vi "SafetySystem.vi"() -> ()   [LabVIEW 2018]
uses:
  <vilib>/Platform/TimedLoop/XDataNode/timing_clust.ctl
  <vilib>/Platform/TimedLoop/XDataNode/nitl_modes.ctl
  <vilib>/Platform/TimedLoop/XDataNode/wakeup.ctl
  <vilib>/Modbus/slave/Create Slave Instance (TCP).vi
  <vilib>/Modbus/slave/Modbus Slave.lvclass
  <vilib>/Platform/TimedLoop/XDataNode/XDataNode.xnode
  <vilib>/Platform/TimedLoop/XDataNode/XDNodeRunTimeDep.lvlib
panel:
  out "SIS-10SDV501":bool
  out "SIS-10SDV502":bool
  out "SIS-10SDV500":bool
  out "SIS-10TI101":dbl
  out "SIS-10AI301":dbl
  out "SIS-10LI202":dbl
  out "SIS-10LI201":dbl
  in  "stop":bool
  out "TX-SIS-BPCS-ARRAY":bool[](array[boolean])
  out "BPCS-SIM-TX-ARRAY":dbl[](array[numeric])
  out "SIM-SIS-RX-ARRAY":dbl[](array[numeric])
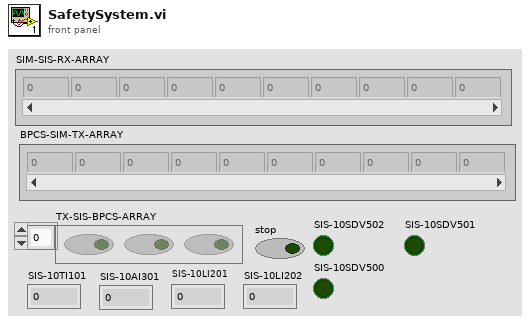
[diagram p1: front panel]
types:
  T1 = typedef "XDNodeRunTimeDep.lvlib/timing_clust.ctl" = cluster{"Expected End [f-1]":u64, "Actual End [f-1]":u64, "Finished Late? [f-1]":bool, "Expected End [i-1]":u64, "Actual End [i-1]":u64, "Finished Late? [i-1]":bool, "Expected Start [i]":u64, "Actual Start [i]":u64, "Expected Start [f]":u64, "Actual Start [f]":u64, "Source Name":string, "Structure Name":string, "Period":i64, "Deadline":i64, "Offset":i64, "Start":i64, "Priority":i32, "Timeout":i32, "Mode":T2, "Wakeup Reason":T3, "Error":errorcluster, "Source Type":string, "Secondary Source Type":string, "Global End Time":u64, "Global Start Time":u64, "Frame Duration":u64, "Iteration Duration":u64, "Assigned CPU":i32, "I/O Scan Engine Mode":u32}
  T2 = typedef "XDNodeRunTimeDep.lvlib/nitl_modes.ctl" = enum32{"No Change", "Process missed periods, maintain original phase", "Discard missed periods, maintain original phase", "Process missed periods, ignore original phase", "Discard missed periods, ignore original phase"}
  T3 = typedef "XDNodeRunTimeDep.lvlib/wakeup.ctl" = enum32{"Normal", "Aborted", "Asynchronous wakeup", "Timing source error", "Timed loop error", "Timeout"}
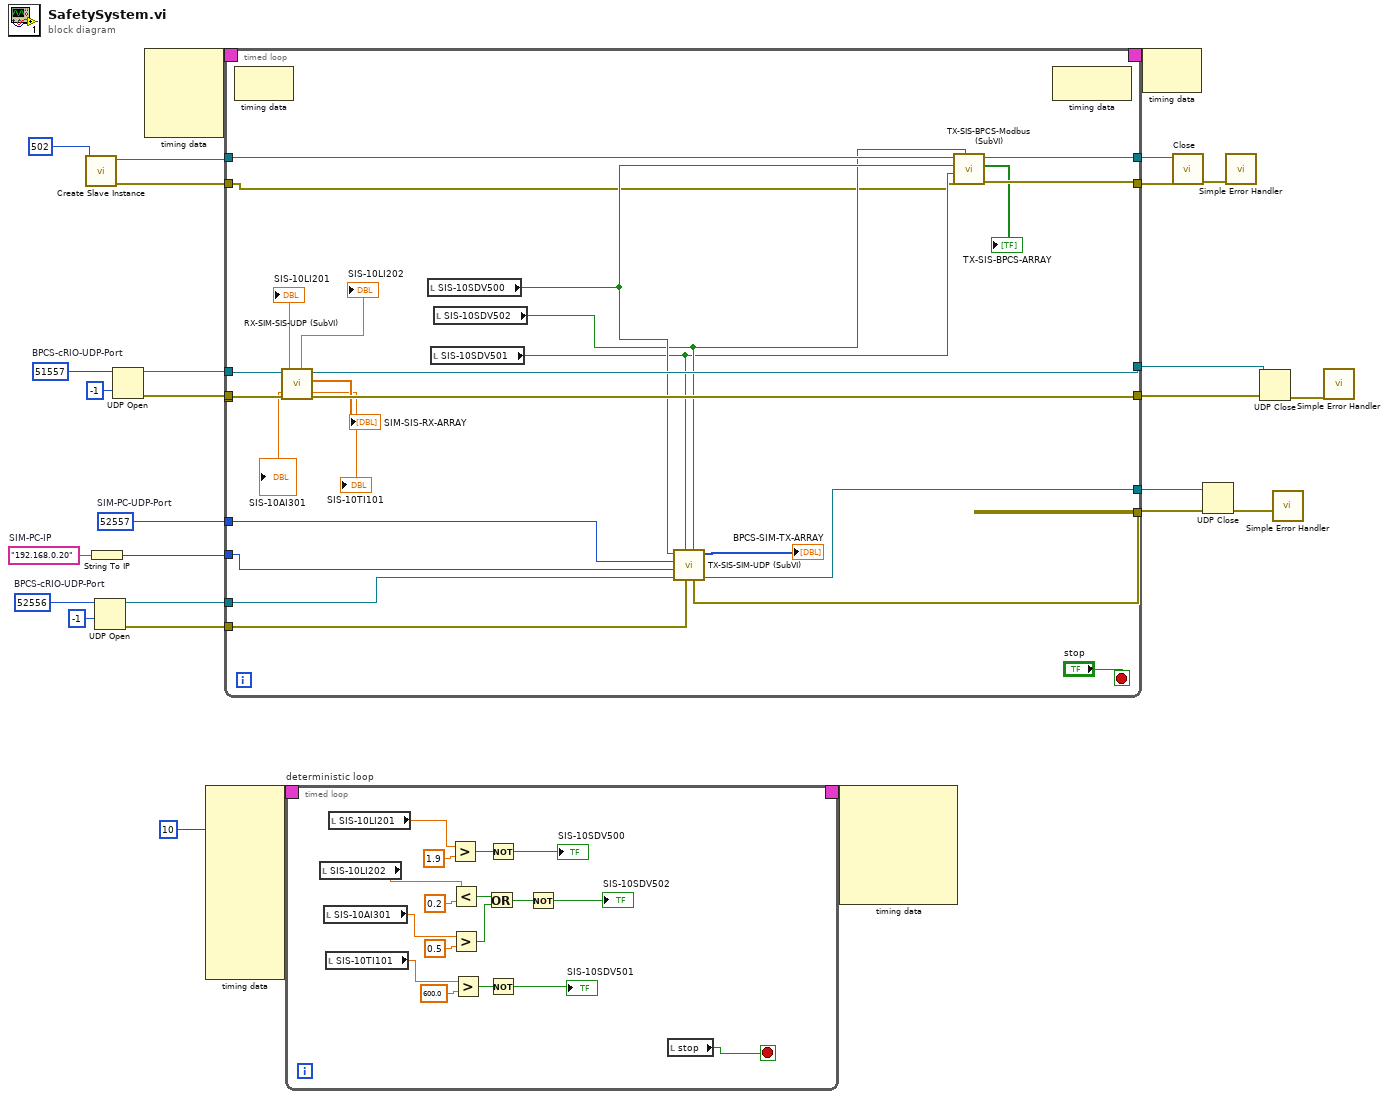
[diagram p0: block diagram]
diagram:
  w18 = u16 52556  # BPCS-cRIO-UDP-Port
  w16 = u16 52557  # SIM-PC-UDP-Port
  w19 = "192.168.0.20"  # SIM-PC-IP
  w25 = u16 51557  # BPCS-cRIO-UDP-Port
  n1 = call-poly <vilib>:"Create Slave Instance.vi"("port (502)"=u16 502) -> ("error out"=w8:errorcluster, "TCP slave instance"=w9:refnum<class "Modbus Slave.lvclass">)  [unwired: 9 in]
  n2 = String To IP(1:w19) -> (0:w15:u32)
  n3 = UDP Open(9:-1 ("timeout ms (25000)"), 11:w18) -> (port=w14:refnum<k16>, 0:w13:errorcluster)  [unwired: 3 in, 1 out]
  n4 = UDP Open(9:-1 ("timeout ms (25000)"), 11:w25) -> (port=w24:refnum<k16>, 0:w23:errorcluster)  [unwired: 3 in, 1 out]
  n5 = node-c288() -> (w28:T1)  [unwired: 4 in]
  n6 = node-c288 ("Input Node")(i64 10 ("Period")) -> (w4:T1)  [unwired: 9 in]
  n7 = timed-loop {
    timing: w28 -> [_]
    timing-out: [_] -> w27
    tunnel: w24 -> [w53]
    tunnel: [w52] -> _
    tunnel: w23 -> [w52]
    tunnel: [w51] -> w21
    tunnel: [w50] -> w20
    tunnel: w16 -> [w40]
    tunnel: w15 -> [w39]
    tunnel: w14 -> [w44]
    tunnel: w13 -> [w43]
    tunnel: [w42] -> w10
    tunnel: [w41] -> w11
    tunnel: w9 -> [w37]
    tunnel: [w36] -> w6
    tunnel: w8 -> [w29]
    tunnel: [w35] -> w5
    stop <- "stop" stop-if-true
    n8 = node-c288() -> ()  [unwired: 1 in, 1 out]
    n9 = call "RX-SIM-SIS-UDP (SubVI).vi"("error in (no error)"=w52, "UDP Network Connection in"=w53) -> ("error out"=w50:errorcluster, "SIM-SIS-RX-ARRAY"=→"SIM-SIS-RX-ARRAY":dbl[], "UDP Network Connection out"=w51:refnum<k16>, "SIS-10TI101"=→"SIS-10TI101":dbl, "SIS-10LI202"=→"SIS-10LI202":dbl, "SIS-10AI301"=→"SIS-10AI301":dbl, "SIS-10LI201"=→"SIS-10LI201":dbl)  [unwired: 3 in]
    n10 = local read "SIS-10SDV500"() -> (w32:bool)
    n11 = local read "SIS-10SDV501"() -> (w30:bool)
    n12 = local read "SIS-10SDV502"() -> (w31:bool)
    n13 = call "TX-SIS-SIM-UDP (SubVI).vi"("SIS-10SDV502"=w31, "error in (no error)"=w43, "SIS-10SDV501"=w30, "UDP Network Connection in"=w44, "SIM-PC-IP"=w39, "SIM-PC-UDP-Port"=w40, "SIS-10SDV500"=w32) -> ("UDP Network Connection out"=w41:refnum<k16>, "BPCS-SIM-TX-ARRAY"=→"BPCS-SIM-TX-ARRAY":i16[], "error out"=w42:errorcluster)  [unwired: 2 in]
    n14 = call "TX-SIS-BPCS-Modbus (SubVI).vi"("SIS-10SDV502"=w31, "error in (no error)"=w29, "SIS-10SDV501"=w30, "SIS-10SDV500"=w32, "Modbus Slave in"=w37) -> ("error out"=w35:errorcluster, "TX-SIS-BPCS-ARRAY"=→"TX-SIS-BPCS-ARRAY":bool[], "Modbus Slave out"=w36:refnum<class "Modbus Slave.lvclass">)  [unwired: 4 in]
    n15 = node-c288() -> ()  [unwired: 1 in, 1 out]
  }
  n16 = timed-loop "deterministic loop" {
    timing: w4 -> [_]
    timing-out: [_] -> w3
    stop <- w56 stop-if-true
    n17 = local read "SIS-10LI202"() -> (w62:dbl)
    n18 = local read "SIS-10AI301"() -> (w61:dbl)
    n19 = local read "SIS-10TI101"() -> (w60:dbl)
    n20 = local read "SIS-10LI201"() -> (w63:dbl)
    n21 = Greater?(x=w63, y=1.9) -> (0:w71:bool)
    n22 = Less?(x=w62, y=0.2) -> (x < y?=w67:bool)
    n23 = Greater?(x=w61, y=0.5) -> (0:w66:bool)
    n24 = Greater?(x=w60, y=600.0) -> (0:w69:bool)
    n25 = Or(x=w67, y=w66) -> (x .or. y?=w65:bool)
    n26 = Not(x=w71) -> (.not. x?=→"SIS-10SDV500":bool)
    n27 = Not(x=w69) -> (.not. x?=→"SIS-10SDV501":bool)
    n28 = Not(x=w65) -> (.not. x?=→"SIS-10SDV502":bool)
    n29 = local read "stop"() -> (w56:bool)
  }
  n30 = node-c288 ("Output Node")(w3) -> ()  [unwired: 6 out]
  n31 = node-c288(w27) -> ()  [unwired: 1 out]
  n32 = call-dynamic "Close.vi"("error in (no error)"=w5, "Modbus slave in"=w6) -> ("error out"=w7:errorcluster)  [unwired: 9 in]
  n33 = UDP Close(connection ID=w11, 8:w10) -> (error out=w12:errorcluster)  [unwired: 1 out]
  n34 = call <vilib>:"Simple Error Handler.vi"("error in (no error)"=w7) -> ()  [unwired: 4 in, 5 out]
  n35 = UDP Close(connection ID=w21, 8:w20) -> (error out=w22:errorcluster)  [unwired: 1 out]
  n36 = call <vilib>:"Simple Error Handler.vi"("error in (no error)"=w12) -> ()  [unwired: 4 in, 5 out]
  n37 = call <vilib>:"Simple Error Handler.vi"("error in (no error)"=w22) -> ()  [unwired: 4 in, 5 out]
